vi "Set camera gain.vi"(8 "Error In":errorcluster, 9 "Gain Boost in":bool, 10 "Gain in":i32, 11 ".NET (Reference)":refnum<k24>) -> (0 "Error Out":errorcluster, 1 "Gain boost out":bool, 2 "Gain out":i32)   [LabVIEW 2017]
uses:
  C:/Program Files/National Instruments/LabVIEW 2017/instr.lib/IDS/ueye.NET/uEyeDotNet.dll
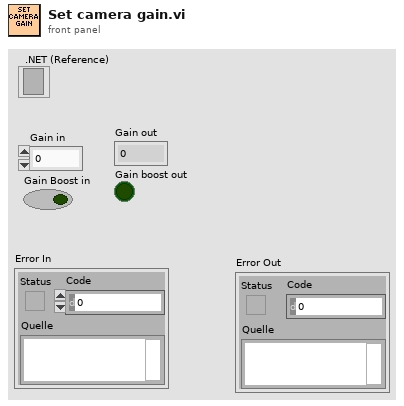
[diagram p1: front panel]
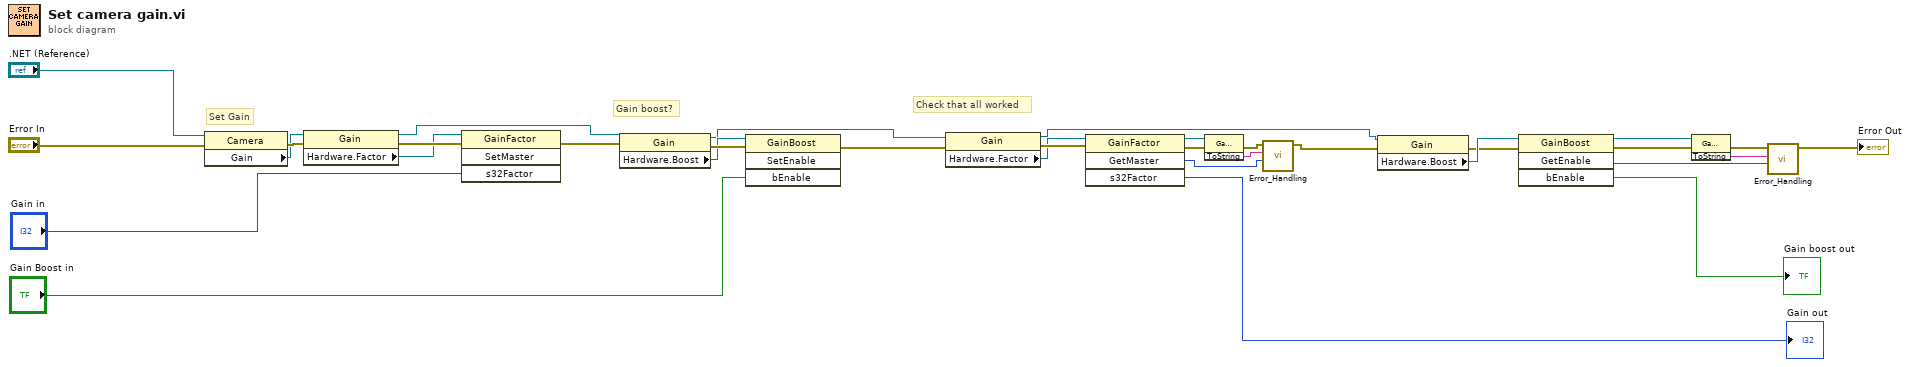
[diagram p0: block diagram]
diagram:
  # "Check that all worked"
  # "Gain boost?"
  # "Set Gain"
  n1 = property class="Camera"(reference=".NET (Reference)", error in="Error In") -> (error out=w30:errorcluster, "Gain"=w27:refnum<k24>)  [unwired: 1 out]
  n2 = property class="Gain"(reference=w27, error in=w30) -> (reference out=w25:refnum<k24>, error out=w31:errorcluster, "Hardware.Factor"=w29:refnum<k24>)
  n3 = invoke class="GainFactor" method="SetMaster"(reference=w29, error in=w31, "s32Factor"="Gain in") -> (error out=w1:errorcluster)  [unwired: 1 in, 3 out]
  n4 = property class="Gain"(reference=w25, error in=w1) -> (reference out=w22:refnum<k24>, error out=w26:errorcluster, "Hardware.Boost"=w24:refnum<k24>)
  n5 = invoke class="GainBoost" method="SetEnable"(reference=w24, error in=w26, "bEnable"="Gain Boost in") -> (error out=w21:errorcluster)  [unwired: 1 in, 3 out]
  n6 = property class="Gain"(reference=w22, error in=w21) -> (reference out=w13:refnum<k24>, error out=w20:errorcluster, "Hardware.Factor"=w19:refnum<k24>)
  n7 = invoke class="GainFactor" method="GetMaster"(reference=w19, error in=w20) -> (reference out=w6:refnum<k24>, error out=w17:errorcluster, "GetMaster"=w15:i32, "s32Factor"=→"Gain out":i32)  [unwired: 2 in]
  n8 = invoke class="GainFactor" method="ToString"(reference=w6, error in=w17) -> (error out=w14:errorcluster, "ToString"=w16:string)  [unwired: 1 in, 1 out]
  n9 = call <instrlib>:"Error_Handling.vi"("Error Code"=w15, "Error String"=w16, "Error In"=w14) -> ("Error Out"=w3:errorcluster)  [unwired: 8 in]
  n10 = property class="Gain"(reference=w13, error in=w3) -> (error out=w2:errorcluster, "Hardware.Boost"=w12:refnum<k24>)  [unwired: 1 out]
  n11 = invoke class="GainBoost" method="GetEnable"(reference=w12, error in=w2) -> (reference out=w8:refnum<k24>, error out=w7:errorcluster, "GetEnable"=w5:i32, "bEnable"=→"Gain boost out":bool)  [unwired: 2 in]
  n12 = invoke class="GainBoost" method="ToString"(reference=w8, error in=w7) -> (error out=w9:errorcluster, "ToString"=w10:string)  [unwired: 1 in, 1 out]
  n13 = call <instrlib>:"Error_Handling.vi"("Error Code"=w5, "Error String"=w10, "Error In"=w9) -> ("Error Out"=→"Error Out":errorcluster)  [unwired: 8 in]
